vi "FPGAcode.vi"() -> ()   [LabVIEW 2021]
uses:
  <vilib>/rvi/eio/common/nirviEmuTemplateMethod_errors.vi
  <vilib>/rvi/Emulation/niFpgaGetClockAttributes.vi
  <vilib>/rvi/Emulation/niFpgaSctlEmulationGetInTimedLoop.vi
  <vilib>/rvi/Emulation/niFpgaEmulationReportErrorSimple.vi
  <vilib>/rvi/Emulation/niFpgaCriticalErrorInLSC.vi
  <vilib>/eio/EIONode/EIONode.xnode
panel:
  in  "LED0":bool
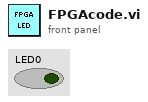
[diagram p1: front panel]
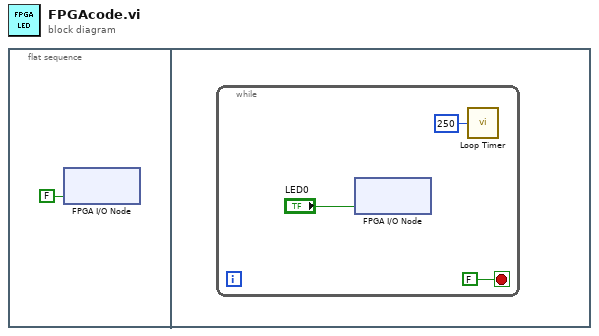
[diagram p0: block diagram]
diagram:
  n1 = flat-sequence {
    frame #0 {
      n2 = xnode "FPGA I/O Node"("LED0"=FALSE) -> ()  [unwired: 1 in, 1 out]
    }
    frame #1 {
      n3 = while {
        stop <- FALSE stop-if-true
        n4 = xnode "FPGA I/O Node"("LED0"="LED0") -> ()  [unwired: 1 in, 1 out]
        n5 = call "Loop Timer"("Count(mSec)"=u32 250) -> ()  [unwired: 1 out]
      }
    }
  }
